vi "Stop all live.vi"(7 "Error In":errorcluster, 10 "Camera cluster":T1) -> (0 "Error Out":errorcluster)   [LabVIEW 2017]
uses:
  C:/Program Files/National Instruments/LabVIEW 2017/instr.lib/IDS/ueye.NET/uEyeDotNet.dll
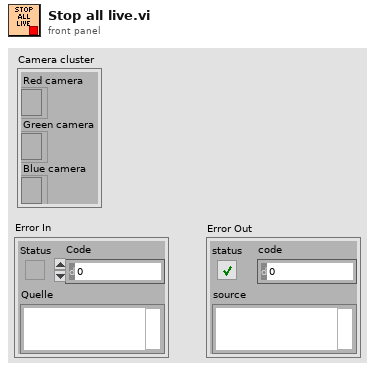
[diagram p1: front panel]
types:
  T1 = cluster{"Red camera":refnum<k24>, "Green camera":refnum<k24>, "Blue camera":refnum<k24>}
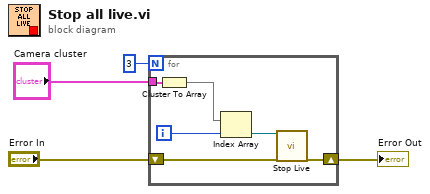
[diagram p0: block diagram]
diagram:
  n1 = for {
    N: 3 -> [_]
    tunnel: "Camera cluster" -> [w9]
    shift-right: [w7] -> w2
    shift-left: "Error In" -> [w6]
    i -> [w5]
    n2 = Cluster To Array(cluster=w9) -> (array=w10:refnum<k24>[])
    n3 = Index Array(array=w10, index=w5) -> (element=w8:refnum<k24>)
    n4 = call "Stop Live.vi"("Camera reference in"=w8, "Error In"=w6) -> ("Error Out"=w7:errorcluster)  [unwired: 16 in, 1 out]
  }
  "Error Out" <- w2
